vi "4.3.vi"() -> ()   [LabVIEW 2017]
panel:
  out "a":dbl
  in  "x":dbl
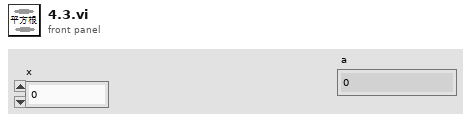
[diagram p1: front panel]
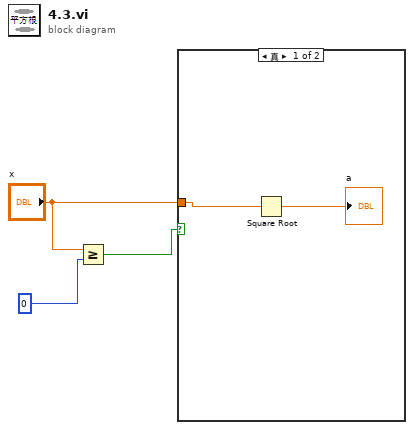
[diagram p0: block diagram]
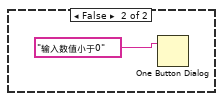
[diagram p2: hidden frame]
diagram:
  n1 = Greater Or Equal?(x="x", y=0) -> (x >= y?=w2:bool)
  n2 = case shown="真" w2 {
    tunnel: "x" -> [w5 _]
    frame True {
      n3 = Square Root(x=w5) -> (sqrt(x)=→"a":dbl)
    }
    frame False {
      n4 = One Button Dialog(message="输入数值小于0") -> ()  [unwired: 1 in, 1 out]
    }
  }
